vi "Write system.vi"(8 "error in (no error)":errorcluster, 10 "system":string, 11 "channel config object in":refnum<class "channel configuration.lvclass">) -> (0 "error out":errorcluster, 3 "channel config object out":refnum<class "channel configuration.lvclass">)   [LabVIEW 2013, in "channel configuration.lvclass"]
uses:
  channel configuration.lvclass
  channel configuration.lvclass/channel configuration.ctl
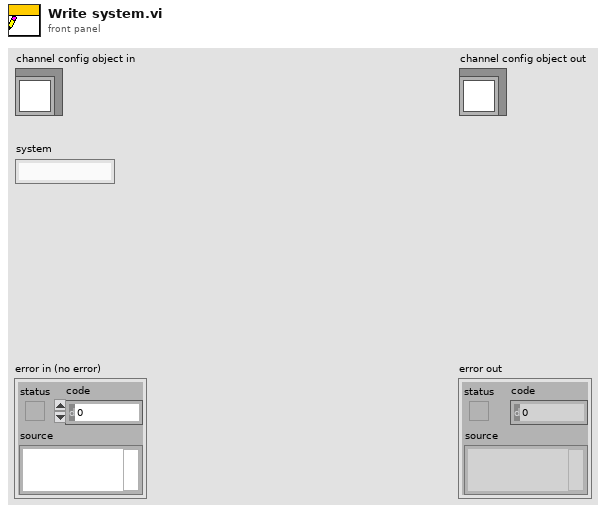
[diagram p1: front panel]
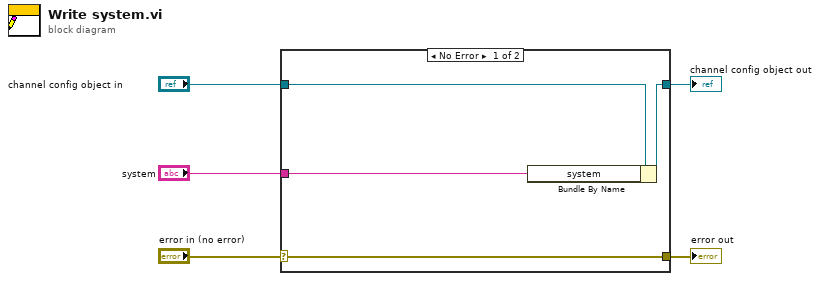
[diagram p0: block diagram]
diagram:
  n1 = case shown="No Error" "error in (no error)" {
    selector: "error in (no error)" -> [w9 w10]
    tunnel: [w9 w10] -> w4
    tunnel: [w7 w11] -> w2
    tunnel: "channel config object in" -> [w8 w11]
    tunnel: "system" -> [w6 _]
    frame No Error {
      n2 = Bundle By Name(cluster=w8, "system"=w6) -> (w7:refnum<class "channel configuration.lvclass">)
    }
    frame Error {
    }
  }
  "error out" <- w4
  "channel config object out" <- w2
